vi "Configure Temperature.vi"(6 "Transducer Type":u16(ring)=1 items=["Thermocouple", "Thermistor", "3-wire RTD", " 4-wire RTD"], 8 "error in (no error)":errorcluster, 9 "NPLC":u16(ring)=1 items=["0.00005", "1", "12", "15"], 10 "Aperture Seconds":dbl, 11 "VISA resource name":refnum<visa-resource-name>) -> (0 "error out":errorcluster, 3 "VISA resource name out":refnum<visa-resource-name>)   [LabVIEW 2018, in "Keithley DMM7512.lvlib"]
doc: "This VI configures the Temperature measurement function parameters like transducer type, NPLC and the aperture setting."
uses:
  <instrlib>/Keithley DMM7512/Keithley DMM7512.lvlib
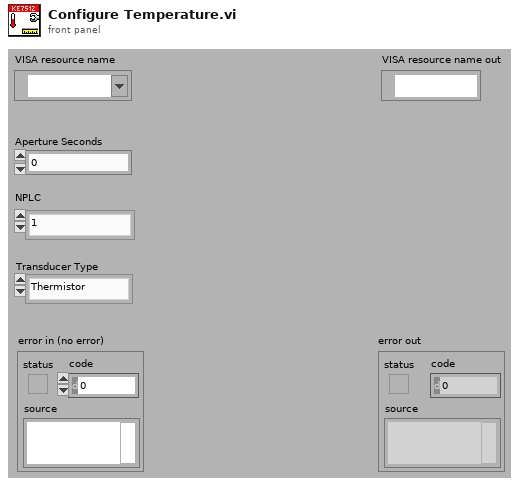
[diagram p1: front panel]
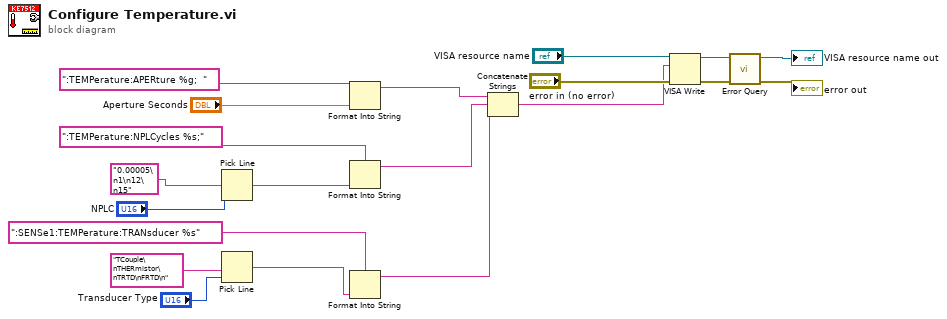
[diagram p0: block diagram]
diagram:
  n1 = Pick Line(multi-line string="0.00005\n1\n12\n15", line index="NPLC") -> (output string=w10:string)  [unwired: 1 in]
  n2 = Pick Line(multi-line string="TCouple\nTHERmistor\nTRTD\nFRTD\n", line index="Transducer Type") -> (output string=w7:string)  [unwired: 1 in]
  n3 = Format Into String(format string=":TEMPerature:APERture %g;  ", "Aperture Seconds") -> (resulting string=w15:string)  [unwired: 2 in, 1 out]
  n4 = Format Into String(format string=":TEMPerature:NPLCycles %s;", w10) -> (resulting string=w14:string)  [unwired: 2 in, 1 out]
  n5 = Format Into String(format string=":SENSe1:TEMPerature:TRANsducer %s", w7) -> (resulting string=w5:string)  [unwired: 2 in, 1 out]
  n6 = Concatenate Strings(w15, w14, w5) -> (w13:string)
  n7 = VISA Write(VISA resource name="VISA resource name", write buffer=w13, error in (no error)="error in (no error)") -> (VISA resource name out=w4:refnum<visa-resource-name>, error out=w3:errorcluster)  [unwired: 1 out]
  n8 = call <instrlib>:"Error Query.vi"("error in (no error)"=w3, "VISA resource name"=w4) -> ("error out"=→"error out":errorcluster, "VISA resource name out"=→"VISA resource name out":refnum<visa-resource-name>)  [unwired: 6 in, 2 out]
